vi "Read Analogue.vi"(8 "error in (no error)":errorcluster, 11 "Chroma190020 HiPOT in":refnum<class "Chroma190020 HiPOT.lvclass">) -> (0 "error out":errorcluster, 2 "Measurements":dbl, 3 "Chroma190020 HiPOT out":refnum<class "Chroma190020 HiPOT.lvclass">)   [LabVIEW 2019, in "Concrete.lvlib" / "Chroma190020 HiPOT.lvclass"]
uses:
  Chroma190020 HiPOT.lvclass
  Chroma190020 HiPOT.lvclass/Chroma190020 HiPOT.ctl
  Harware Abstraction/Analog In/Analog In.lvclass
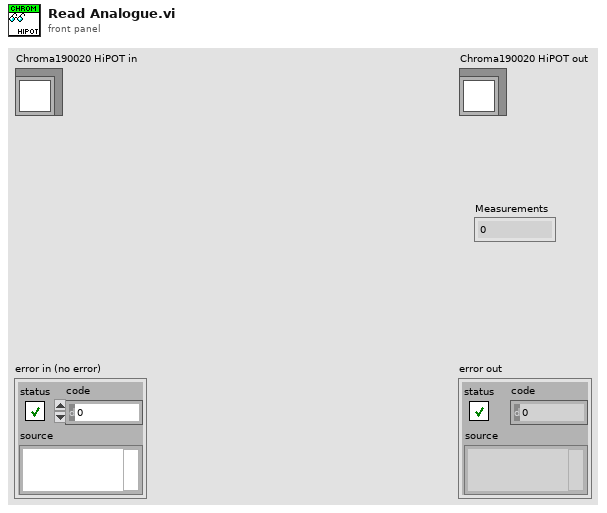
[diagram p1: front panel]
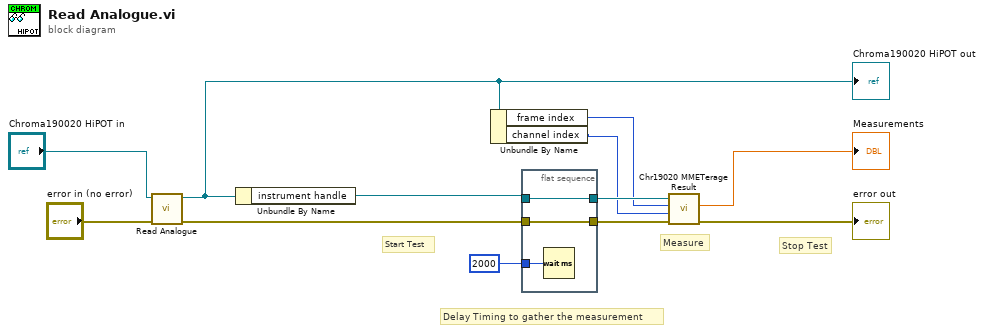
[diagram p0: block diagram]
diagram:
  # "Delay Timing to gather the measurement"
  # "Stop Test"
  # "Start Test"
  # "Measure"
  n1 = call-parent "Read Analogue.vi"("error in (no error)"="error in (no error)", "PS in"="Chroma190020 HiPOT in") -> ("error out"=w3:errorcluster, "PS out"=w7:refnum<class "Chroma190020 HiPOT.lvclass">)  [unwired: 7 in, 1 out]
  "Chroma190020 HiPOT out" <- w7
  n2 = Unbundle By Name(w7) -> ("instrument handle"=w4:refnum<k15>)
  n3 = Unbundle By Name(w7) -> ("frame index"=w6:i32, "channel index"=w5:i32)
  n4 = flat-sequence {
    tunnel: u32 2000 -> [w13]
    tunnel: [w15] -> w2
    tunnel: w3 -> [w15]
    tunnel: [w14] -> w9
    tunnel: w4 -> [w14]
    frame #0 {
      n5 = Wait (ms)(milliseconds to wait=w13) -> ()  [unwired: 1 out]
    }
  }
  n6 = call <instrlib>:"Chr19020 MMETerage Result.vi"("error in (no error)"=w2, "channel index"=w5, "frame index"=w6, "instrument handle"=w9) -> ("error out"=→"error out":errorcluster, "return value"=→"Measurements":dbl)  [unwired: 5 in, 1 out]
